vi "Get Name Chain.vi"(11 "Window Name":string="123_456_789") -> (2 "Module Name":string, 3 "Name Chain":string[](array[string]))   [LabVIEW 2018, in "MainInterface.lvlib" / "User Interface.lvclass"]
uses:
  User Interface.lvclass
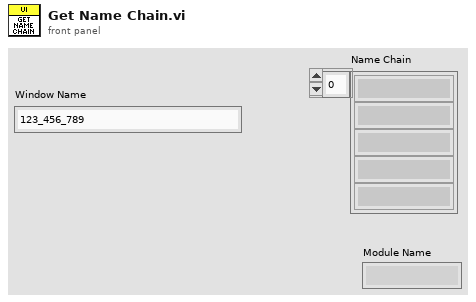
[diagram p1: front panel]
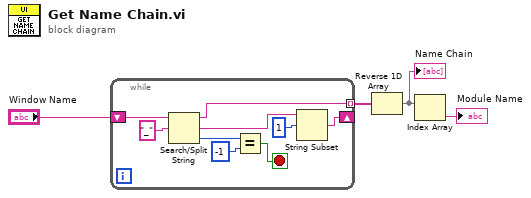
[diagram p0: block diagram]
diagram:
  n1 = while {
    shift-right: [w9] -> _
    shift-left: "Window Name" -> [w13]
    tunnel: [w8] -> w3 mode=indexing
    stop <- w5 stop-if-true
    n2 = Search/Split String(string=w13, search string/char (-)="_" ("搜索字符串/字符(-)")) -> (substring before match=w8:string, match + rest of string=w11:string, offset of match=w7:i32)  [unwired: 1 in]
    n3 = Equal?(x=w7, y=-1) -> (x = y?=w5:bool)
    n4 = String Subset(string=w11, offset (0)=1 ("偏移量(0)")) -> (substring=w9:string)  [unwired: 1 in]
  }
  n5 = Reverse 1D Array(array=w3) -> (reversed array=w2:string[])
  "Name Chain" <- w2
  n6 = Index Array(array=w2) -> (element=→"Module Name":string)  [unwired: 1 in]
